vi "DE_PARTICLE_REPORT_A_MATCHES(SubVI).vi"(1 "Particle Reports (Pixels)":T3(array[cluster]) {"Orientation" format="%.2f"; "Dimensions"."Height" format="%.2f"; "Dimensions"."Width" format="%.2f"; "Center of Mass"."Y" format="%.2f"; "Center of Mass"."X" format="%.2f"; "Bounding Rect"."Bottom" format="%.2f"; "Bounding Rect"."Right" format="%.2f"; "Bounding Rect"."Top" format="%.2f"; "Bounding Rect"."Left" format="%.2f"; "Number of Holes" format="%.2f"; "Area" format="%.2f"}) -> (0 "Matches":T2(array[cluster]) {"Bounding Box"."y" format="%.2f"; "Bounding Box"."x" format="%.2f"; "Position"."y" format="%.2f"; "Position"."x" format="%.2f"; "Score" format="%.2f"; "Scale" format="%.2f"; "Angle" format="%.2f"})   [LabVIEW 2011]
doc: "cambia DE SHAPE REPORT A MATCHES, para poder en encajar los datos de shape de global rectangle a bunding box y de centroid a position; otros cambias de object Size a Scale, angle ninguno (360 defecto), Score a Score."
panel:
  in  "?":T1 {"Bounding Box"."y" format="%.2f"; "Bounding Box"."x" format="%.2f"; "Position"."y" format="%.2f"; "Position"."x" format="%.2f"; "Score" format="%.2f"; "Scale" format="%.2f"; "Angle" format="%.2f"}
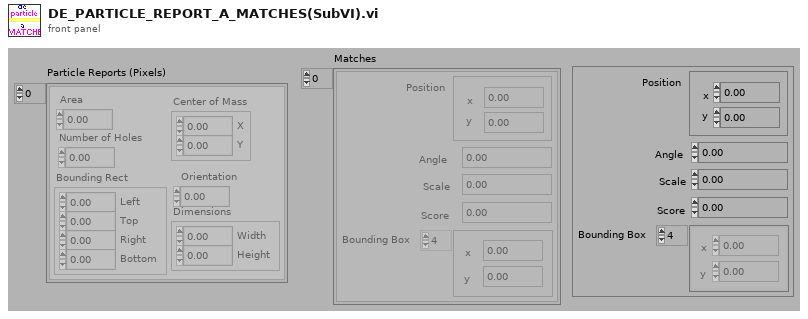
[diagram p1: front panel]
types:
  T1 = cluster{"Position":cluster{"x":sgl, "y":sgl}, "Angle":sgl, "Scale":sgl, "Score":sgl, "Bounding Box":cluster{"x":sgl, "y":sgl}[]}
  T2 = cluster{"Position":cluster{"x":sgl, "y":sgl}, "Angle":sgl, "Scale":sgl, "Score":sgl, "Bounding Box":cluster{"x":sgl, "y":sgl}[]}[]
  T3 = cluster{"Area":dbl, "Number of Holes":dbl, "Bounding Rect":cluster{"Left":dbl, "Top":dbl, "Right":dbl, "Bottom":dbl}, "Center of Mass":cluster{"X":dbl, "Y":dbl}, "Orientation":dbl, "Dimensions":cluster{"Width":dbl, "Height":dbl}}[]
  T4 = cluster{"Left":dbl, "Top":dbl, "Right":dbl, "Bottom":dbl}
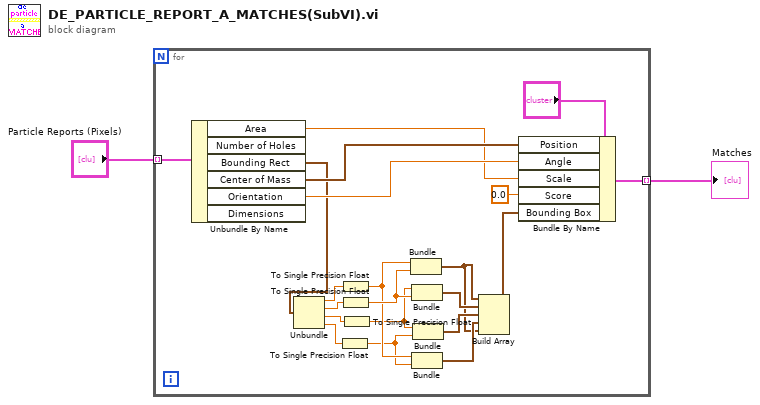
[diagram p0: block diagram]
diagram:
  n1 = for {
    tunnel: "Particle Reports (Pixels)" -> [w23] mode=indexing
    tunnel: [w22] -> w1 mode=indexing
    n2 = Unbundle By Name(w23) -> ("Area"=w19:dbl, "Bounding Rect"=w4:T4, "Center of Mass"=w21:cluster{"X":dbl, "Y":dbl}, "Orientation"=w20:dbl)  [unwired: 2 out]
    n3 = Unbundle(w4) -> ("Left"=w15:dbl, "Top"=w16:dbl, "Right"=w17:dbl, "Bottom"=w14:dbl)
    n4 = To Single Precision Float(number=w14) -> (single precision float=w11:sgl)
    n5 = To Single Precision Float(number=w15) -> (single precision float=w12:sgl)
    n6 = To Single Precision Float(number=w16) -> (single precision float=w13:sgl)
    n7 = To Single Precision Float(number=w17) -> (single precision float=w10:sgl)
    n8 = Bundle(w12, w13) -> (w6:cluster{sgl, sgl})  [unwired: 1 out]
    n9 = Bundle(w10, w13) -> (w9:cluster{sgl, sgl})  [unwired: 1 out]
    n10 = Bundle(w12, w11) -> (w7:cluster{sgl, sgl})  [unwired: 1 out]
    n11 = Bundle(w10, w11) -> (w8:cluster{sgl, sgl})  [unwired: 1 out]
    n12 = Build Array(w6, w9, w8, w7, w6) -> (w5:cluster{sgl, sgl}[])
    n13 = Bundle By Name(cluster="?", "Position"=w21, "Angle"=w20, "Scale"=w19, "Score"=sgl 0.0, "Bounding Box"=w5) -> (w22:T1)
  }
  "Matches" <- w1
